vi "Read Parent Class Info.vi"(8 "error in (no error)":errorcluster) -> (0 "error out":errorcluster, 1 "Class Names":string[](array[string]), 2 "Library Versions":T1(array[cluster]), 3 "Private Data Clusters":variant[](array[variant]))   [LabVIEW 2017, in "TestLibrary.lvlib"]
uses:
  TestLibrary.lvlib
  ParentClass/ParentClass.lvclass
  Composition/Composition.lvlib
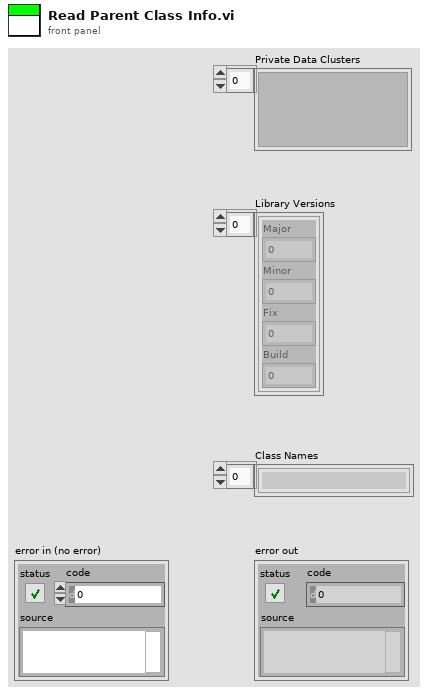
[diagram p1: front panel]
types:
  T1 = cluster{"Major":u16, "Minor":u16, "Fix":u16, "Build":u16}[]
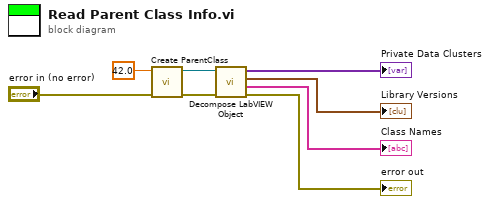
[diagram p0: block diagram]
diagram:
  n1 = call "Create ParentClass.vi"("error in (no error)"="error in (no error)", "Numeric"=42.0) -> ("error out"=w6:errorcluster, "ParentClass"=w7:refnum<class "ParentClass.lvclass">)  [unwired: 8 in]
  n2 = call "Decompose LabVIEW Object.vi"("error in (no error)"=w6, "LabVIEW Object"=w7) -> ("error out"=→"error out":errorcluster, "Class Names"=→"Class Names":string[], "Library Versions"=→"Library Versions":T1, "Private Data Clusters"=→"Private Data Clusters":variant[])  [unwired: 6 in]
